vi "RPM Direction.vi"(11 "Data":dbl) -> (3 "Dataout":string)   [LabVIEW 2022 SP3]
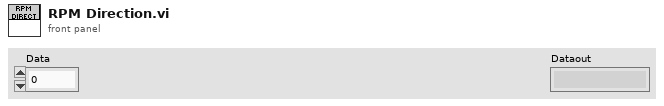
[diagram p1: front panel]
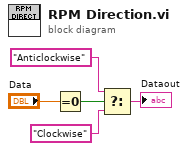
[diagram p0: block diagram]
diagram:
  n1 = Equal To 0?(x="Data") -> (x = 0?=w4:bool)
  n2 = Select(t="Anticlockwise", s=w4, f="Clockwise") -> (s? t:f=→"Dataout":string)
